vi "Hybrid PS control Global.vi"() -> ()   [LabVIEW 2024]
panel:
  in  "User Control":bool
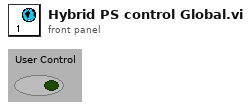
[diagram p1: front panel]
diagram:
